vi "Test MQTT-3.1.3-6.vi"(8 "error in (no error)":errorcluster, 11 "Connection Config":refnum<class "Connection.lvclass">) -> (0 "error out":errorcluster, 3 "Connection Config dup":refnum<class "Connection.lvclass">)   [LabVIEW 2013]
uses:
  <vilib>/LabVIEW Open Source Project/MQTT Connection/MQTT_Connection/Connection/Connection.lvclass
  <vilib>/LabVIEW Open Source Project/MQTT Control Packets/Control Packets/CONNACK/Connect Return Code -- enum.ctl
  <vilib>/LabVIEW Open Source Project/MQTT Control Packets/Control Packets/CONNECT/ConnectFlags -- cluster.ctl
  <vilib>/addons/_JKI Toolkits/Caraya/classes/Test/Test.lvclass
  <vilib>/LabVIEW Open Source Project/MQTT Control Packets/Control Packets/CONNACK/CONNACK.lvclass
  <vilib>/addons/_JKI Toolkits/Caraya/classes/Assert/Assert.lvclass
  <vilib>/LabVIEW Open Source Project/MQTT Client/Client class/Client.lvclass
  <vilib>/LabVIEW Open Source Project/MQTT Control Packets/Control Packets/CONNECT/CONNECT.lvclass
  <vilib>/LabVIEW Open Source Project/MQTT Connection/MQTT_Base/Base Class/MQTT_Base.lvclass
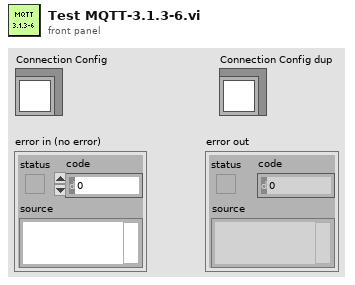
[diagram p1: front panel]
types:
  T1 = typedef "MQTT_Control_Packets.lvlib/CONNECT.lvclass/ConnectFlags -- cluster.ctl" = cluster{"Reserved":bool, "Clean Session":bool, "Will Flag":bool, "Will QoS 1":bool, "Will QoS 2":bool, "Will Retain":bool, "Password Flag":bool, "User Name Flag":bool}
  T2 = typedef "MQTT_Control_Packets.lvlib/CONNACK.lvclass/Connect Return Code -- enum.ctl" = enum16{"Connection accepted", "Unacceptable protocol version", "Identifier Rejected", "Server Unavailable", "Bad Username or Password", "Not Authorized"}
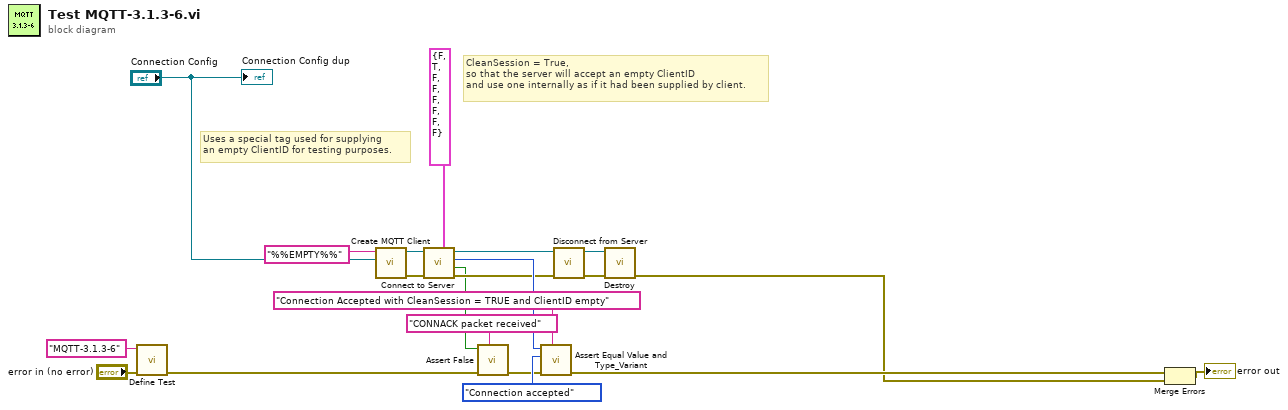
[diagram p0: block diagram]
diagram:
  # "CleanSession = True,\nso that the server will accept an empty ClientID\nand use one internally as if it had been supplied by client."
  # "Uses a special tag used for supplying\nan empty ClientID for testing purposes."
  n1 = call <vilib>:"Define Test.vi"("error in (no error)"="error in (no error)", "Label (VI Title)"="MQTT-3.1.3-6") -> ("error out"=w6:errorcluster)  [unwired: 9 in]
  n2 = call <vilib>:"Create MQTT Client.vi"("Connection Configuration"="Connection Config", "ID (empty:generate new)"="%%EMPTY%%" ("Client ID (empty: generate new)")) -> ("error out"=w11:errorcluster, "Client out"=w12:refnum<class "Client.lvclass">)  [unwired: 8 in]
  n3 = call <vilib>:"Connect to Server.vi"("Connect Flags"=T1 {"Reserved"=FALSE, "Clean Session"=TRUE, "Will Flag"=FALSE, "Will QoS 1"=FALSE, "Will QoS 2"=FALSE, "Will Retain"=FALSE, "Password Flag"=FALSE, "User Name Flag"=FALSE}, "error in (no error)"=w11, "Client in"=w12) -> ("error out"=w8:errorcluster, "timed out"=w7:bool, "Return Code"=w10:T2, "Client out"=w9:refnum<class "Client.lvclass">)  [unwired: 5 in]
  n4 = call <vilib>:"Assert False.vi"("Label"="CONNACK packet received", "error in (no error)"=w6, "False?"=w7) -> ("error out"=w15:errorcluster)  [unwired: 8 in]
  n5 = call <vilib>:"Assert Equal Value and Type_Variant.vi"("Label"="Connection Accepted with CleanSession = TRUE and ClientID empty", "error in (no error)"=w15, "Y"=Connect_Return_Code_--_enum."Connection accepted" ("Return Code"), "X"=w10) -> ("error out"=w20:errorcluster)  [unwired: 7 in]
  n6 = call <vilib>:"Disconnect from Server.vi"("error in (no error)"=w8, "Client in"=w9) -> ("error out"=w4:errorcluster, "Client out"=w2:refnum<class "Client.lvclass">)  [unwired: 7 in, 1 out]
  n7 = call <vilib>:"Destroy.vi"("error in (no error)"=w4, "MQTT_Base in"=w2) -> ("error out"=w3:errorcluster)  [unwired: 8 in, 1 out]
  n8 = Merge Errors(w20, w3) -> (→"error out":errorcluster)
  "Connection Config dup" <- "Connection Config"
